vi "DLL Retcode to VI Errcode.vi"(8 "error in (no error)":errorcluster, 11 "DLL Retcode":i32 format="%x") -> (0 "error out":errorcluster, 3 "VI Errcode":i32 format="%x")   [LabVIEW 2013, in "Keyence LK-G5000.lvlib"]
uses:
  <instrlib>/Keyence LK-G5000/Keyence LK-G5000.lvlib
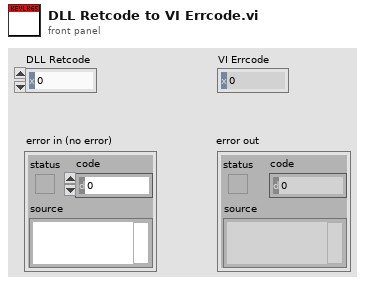
[diagram p1: front panel]
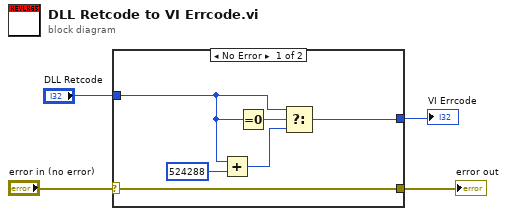
[diagram p0: block diagram]
diagram:
  n1 = case shown="No Error" "error in (no error)" {
    selector: "error in (no error)" -> [w7 w11]
    tunnel: [w7 w11] -> w3
    tunnel: "DLL Retcode" -> [w6 w12]
    tunnel: [w5 w12] -> w1
    frame No Error {
      n2 = Add(x=w6, y=524288) -> (x+y=w8:i32)
      n3 = Equal To 0?(x=w6) -> (x = 0?=w10:bool)
      n4 = Select(t=w6, s=w10, f=w8) -> (s? t:f=w5:i32)
    }
    frame Error {
    }
  }
  "error out" <- w3
  "VI Errcode" <- w1
